vi "AO.Write.vi"(8 "error in (no error)":errorcluster, 11 "AO Data":cluster{"AO Name":string, "AO Value":variant}[](array[cluster])) -> (0 "error out":errorcluster)   [LabVIEW 2019]
doc: "Writes an array of Analog Outputs to hardware, where \"AO Name\" is the name of the channel and \"AO Value\" is the value to write."
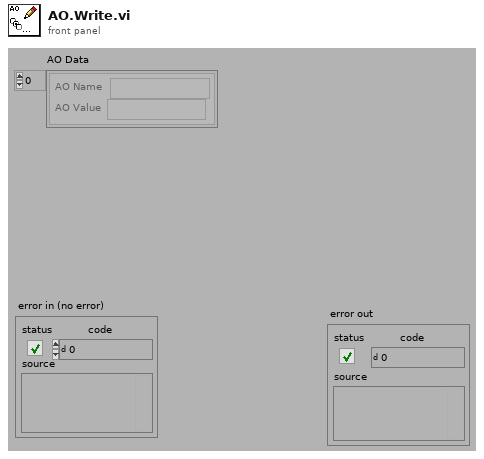
[diagram p1: front panel]
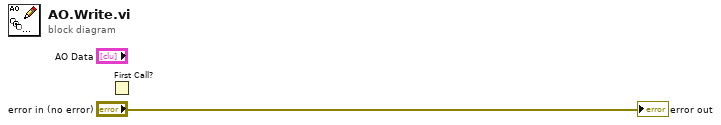
[diagram p0: block diagram]
diagram:
  n1 = First Call?() -> ()  [unwired: 1 out]
  "error out" <- "error in (no error)"
